vi "Draw Path.vi"(8 "error in (no error)":errorcluster, 11 "WayPoints":cluster{sgl, sgl}[](array[cluster])=[{0.5, 0.5}, {0.5, 1.0}, {0.5, 1.5}, {0.5, 2.0}, {0.5, 2.5}, {0.5, 3.0}, {0.79999995, 3.4}, {1.2, 3.7}, {1.7, 3.7}, {2.1, 4.0}, {2.4, 4.4}, {2.7, 4.8}, {3.0, 5.2}, {3.4, 5.5}, {3.9, 5.5}, {4.4, 5.5}, {4.8, 5.8}, {5.3, 5.8}, {5.7, 5.5}, {5.7, 5.0}, {5.7, 4.5}, {5.4, 4.1}, {5.0, 3.8}, {4.7, 3.4}, {4.4, 3.0}, {4.1, 2.6}, {3.8, 2.2}, {3.8, 1.7}, {3.8, 1.2}, {4.1, 0.79999995}, {4.5, 0.5}, {5.0, 0.5}, {5.4, 0.79999995}]) -> (0 "error out":errorcluster)   [LabVIEW 2017]
uses:
  <vilib>/picture/3D Picture Control/Object/Create Object (name).vi
  <vilib>/picture/3D Picture Control/NI_3D Picture Control.lvlib
  <vilib>/robotics/Simulator/NI_Robotics_Simulator.lvlib
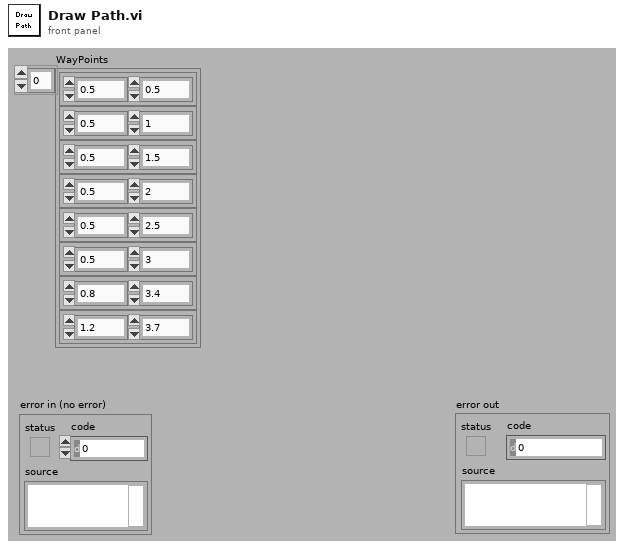
[diagram p1: front panel]
types:
  T1 = cluster{"Red":sgl, "Green":sgl, "Blue":sgl, "Alpha":sgl}
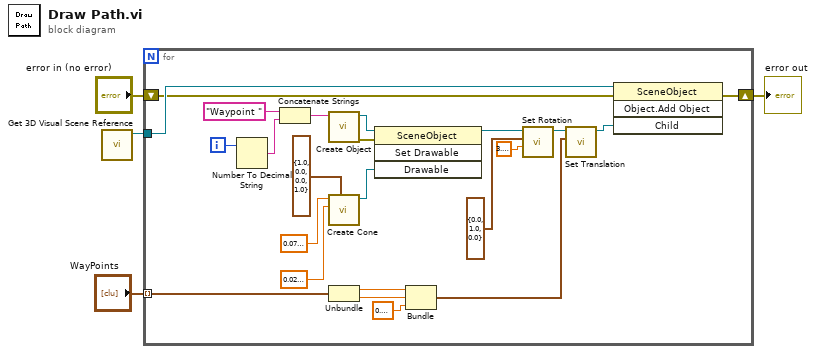
[diagram p0: block diagram]
diagram:
  n1 = call <vilib>:"Get 3D Visual Scene Reference.vi"() -> ("scene ref"=w1:refnum<vi>)  [unwired: 10 in, 1 out]
  n2 = for {
    tunnel: "WayPoints" -> [w13] mode=indexing
    tunnel: w1 -> [w17]
    shift-right: [w5] -> w4
    shift-left: "error in (no error)" -> [w6]
    i -> [w20]
    n3 = Number To Decimal String(number=w20) -> (decimal integer string=w19:string)  [unwired: 1 in]
    n4 = Concatenate Strings("Waypoint " ("string"), w19) -> (w21:string)
    n5 = call-poly <vilib>:"Create Object.vi"("Name"=w21) -> ("error out"=w23:errorcluster, "Scene:New Object"=w24:refnum<vi>)  [unwired: 9 in]
    n6 = call <vilib>:"Create Cone.vi"("Color"=T1 {"Red"=1.0, "Green"=0.0, "Blue"=0.0, "Alpha"=1.0}, "Radius"=sgl 0.03, "Height"=sgl 0.07) -> ("New Cone Refnum"=w18:refnum<vi>)  [unwired: 7 in, 1 out]
    n7 = Unbundle(w13) -> (w8:sgl, w7:sgl)
    n8 = invoke class="SceneObject" method="Set Drawable"(reference=w24, error in=w23, "Drawable"=w18) -> (reference out=w15:refnum<vi>)  [unwired: 1 in, 3 out]
    n9 = Bundle(w8, w7, "Axis:Vel"=sgl 0.1) -> (w11:cluster{sgl, sgl, "Axis:Vel":sgl})  [unwired: 1 in]
    n10 = call <vilib>:"Set Rotation.vi"("Angle"=3.141592653589793, "Axis"=cluster{"X":sgl, "Y":sgl, "Z":sgl} {"X"=0.0, "Y"=1.0, "Z"=0.0}, "Scene Object"=w15) -> ("Rotated Scene Object"=w14:refnum<vi>)  [unwired: 7 in, 1 out]
    n11 = call <vilib>:"Set Translation.vi"("Translation"=w11, "Scene Object"=w14) -> ("Translated Object"=w10:refnum<vi>)  [unwired: 8 in, 1 out]
    n12 = invoke class="SceneObject" method="Object.Add Object"(reference=w17, error in=w6, "Child"=w10) -> (error out=w5:errorcluster)  [unwired: 1 in, 3 out]
  }
  "error out" <- w4
